vi "Servo status changed.vi"(10 "Status before":T1, 11 "Status now":T1) -> (2 "Changed?":bool)   [LabVIEW 2017]
uses:
  ctl/Servo over status.ctl
  ctl/Servo status variable.ctl
  ctl/Servo status constants.ctl
  Servo drive module.lvlib
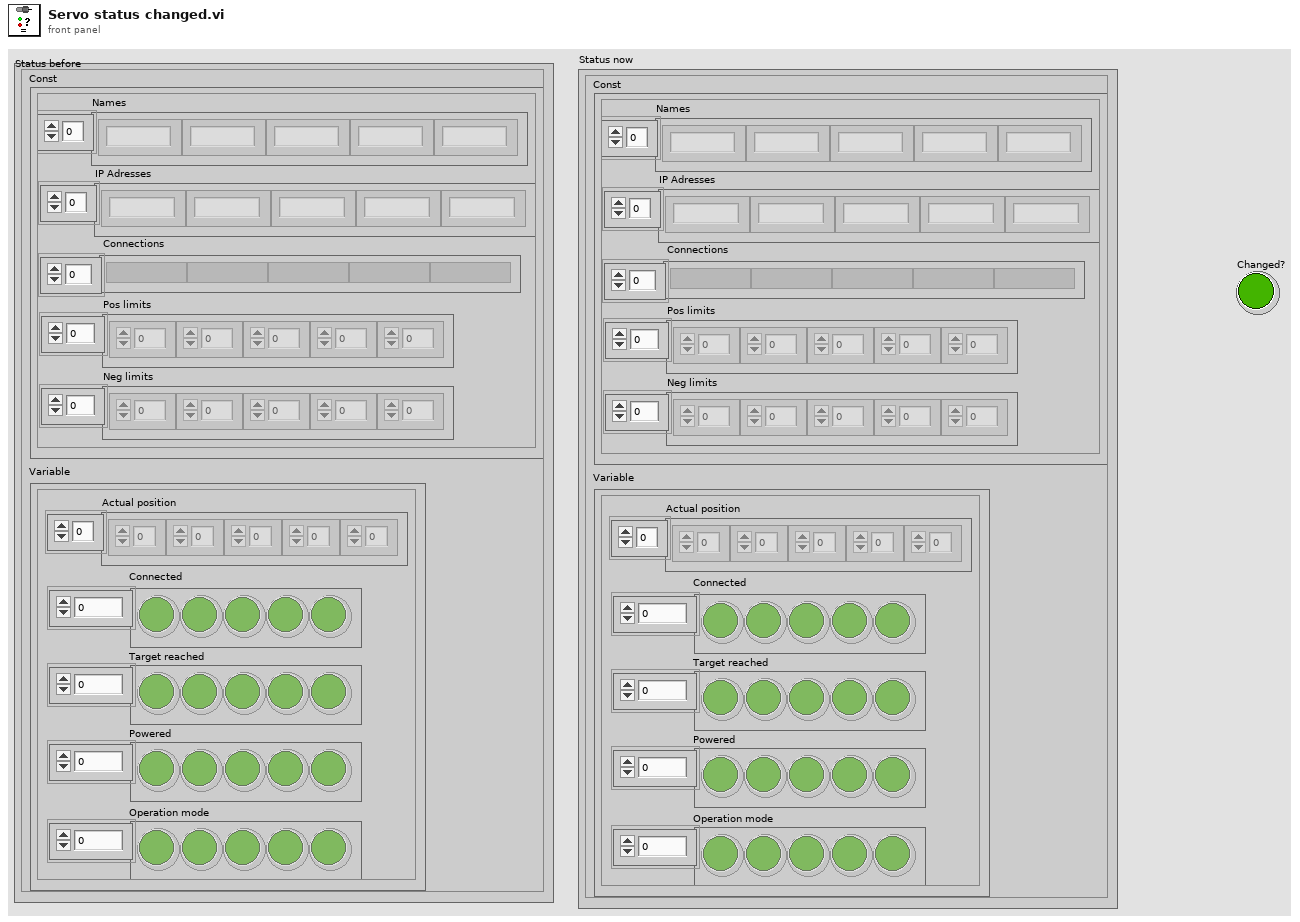
[diagram p1: front panel]
types:
  T1 = typedef "Servo drive module.lvlib/Servo over status.ctl" = cluster{"Variable":T2, "Const":T3}
  T2 = typedef "Servo drive module.lvlib/Servo status variable.ctl" = cluster{"Connected":bool[], "Target reached":bool[], "Powered":bool[], "Actual position":dbl[], "Operation mode":bool[]}
  T3 = typedef "Servo drive module.lvlib/Servo status constants.ctl" = cluster{"IP Adresses":string[], "Names":string[], "Connections":variant[], "Pos limits":dbl[], "Neg limits":dbl[]}
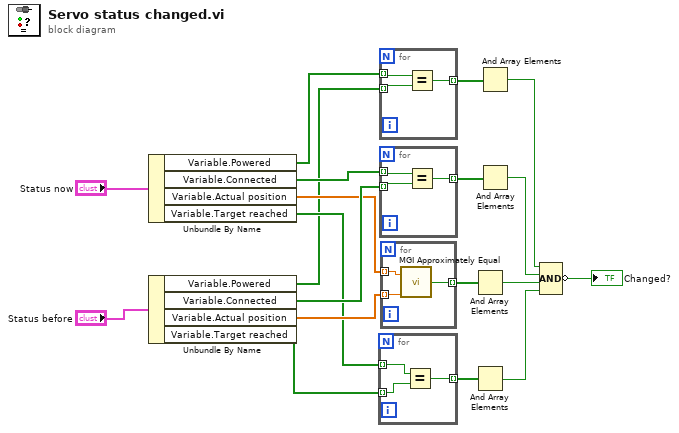
[diagram p0: block diagram]
diagram:
  n1 = Unbundle By Name("Status now") -> ("Variable.Powered"=w3:bool[], "Variable.Connected"=w16:bool[], "Variable.Actual position"=w14:dbl[], "Variable.Target reached"=w12:bool[])
  n2 = Unbundle By Name("Status before") -> ("Variable.Powered"=w2:bool[], "Variable.Connected"=w17:bool[], "Variable.Actual position"=w15:dbl[], "Variable.Target reached"=w13:bool[])
  n3 = for {
    tunnel: w13 -> [w22] mode=indexing
    tunnel: w12 -> [w21] mode=indexing
    tunnel: [w20] -> w11 mode=indexing
    n4 = Equal?(x=w21, y=w22) -> (x = y?=w20:bool)
  }
  n5 = for {
    tunnel: w2 -> [w24] mode=indexing
    tunnel: w3 -> [w25] mode=indexing
    tunnel: [w23] -> w4 mode=indexing
    n6 = Equal?(x=w25, y=w24) -> (x = y?=w23:bool)
  }
  n7 = for {
    tunnel: w17 -> [w27] mode=indexing
    tunnel: w16 -> [w28] mode=indexing
    tunnel: [w26] -> w9 mode=indexing
    n8 = Equal?(x=w28, y=w27) -> (x = y?=w26:bool)
  }
  n9 = for {
    tunnel: w15 -> [w30] mode=indexing
    tunnel: w14 -> [w31] mode=indexing
    tunnel: [w29] -> w10 mode=indexing
    n10 = call <userlib>:"MGI Approximately Equal.vi"("Numeric 2"=w30, "Numeric 1"=w31) -> ("approx = ?"=w29:bool)
  }
  n11 = And Array Elements(Boolean array=w10) -> (logical AND=w7:bool)
  n12 = And Array Elements(Boolean array=w11) -> (logical AND=w6:bool)
  n13 = And Array Elements(Boolean array=w4) -> (logical AND=w1:bool)
  n14 = And Array Elements(Boolean array=w9) -> (logical AND=w8:bool)
  n15 = Compound Arithmetic op=AND(w1, w8, w7, w6) -> (invert →"Changed?":bool)
